vi "Close Excel Application.vi"(8 "error in (no error)":errorcluster, 11 "Excel in":refnum<class "Excel.lvclass">) -> (0 "error out":errorcluster, 3 "Excel out":refnum<class "Excel.lvclass">)   [LabVIEW 2016, in "Excel.lvclass"]
uses:
  Excel.lvclass
  Excel.lvclass/Excel.ctl
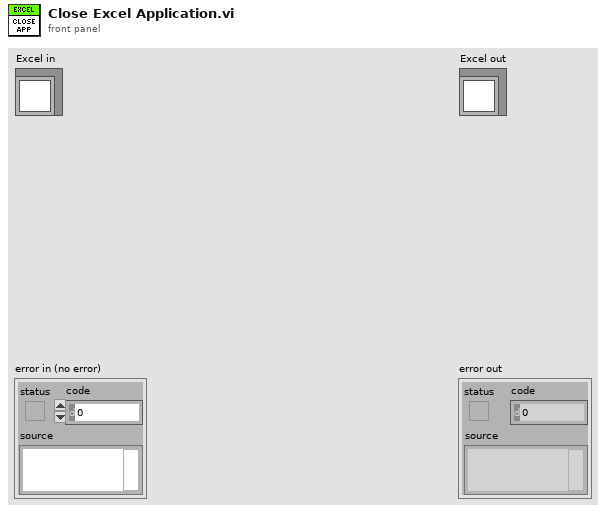
[diagram p1: front panel]
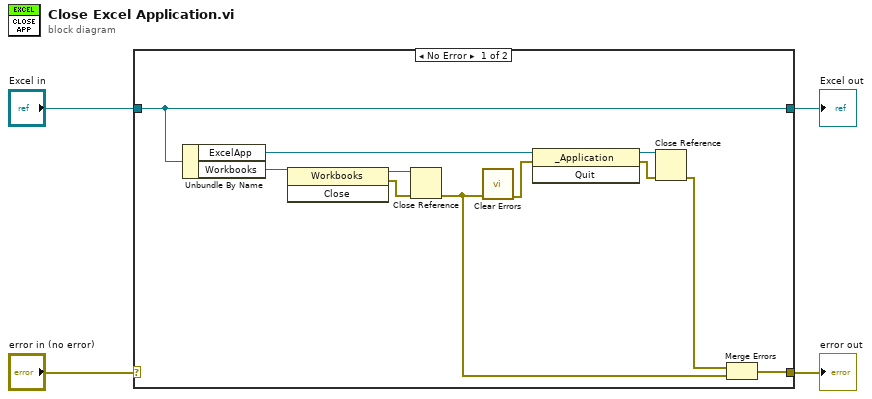
[diagram p0: block diagram]
diagram:
  n1 = case shown="No Error" "error in (no error)" {
    selector: "error in (no error)" -> [_ w17]
    tunnel: [w8 w17] -> w3
    tunnel: [w15 w16] -> w1
    tunnel: "Excel in" -> [w15 w16]
    frame No Error {
      n2 = Unbundle By Name(w15) -> ("ExcelApp"=w11:refnum<k7>, "Workbooks"=w14:refnum<k7>)
      n3 = invoke class="Workbooks" method="Close"(reference=w14) -> (reference out=w13:refnum<k7>, error out=w12:errorcluster)  [unwired: 2 in, 1 out]
      n4 = Close Reference(reference=w13, error in (no error)=w12) -> (error out=w9:errorcluster)
      n5 = call <vilib>:"Clear Errors.vi"("error in (no error)"=w9) -> ("error out"=w10:errorcluster)  [unwired: 5 in, 1 out]
      n6 = invoke class="_Application" method="Quit"(reference=w11, error in=w10) -> (reference out=w6:refnum<k7>, error out=w7:errorcluster)  [unwired: 1 in, 1 out]
      n7 = Close Reference(reference=w6, error in (no error)=w7) -> (error out=w5:errorcluster)
      n8 = Merge Errors(w5, w9) -> (w8:errorcluster)
    }
    frame Error {
    }
  }
  "error out" <- w3
  "Excel out" <- w1
